vi "formate date.vi"(9 "Sepertaor":string, 10 "Input Date":string, 11 "Layout":string(combo)="[MMM-YYYY]") -> (2 "Formatted Date":string)   [LabVIEW 2015]
panel:
  in  "error in (no error)":errorcluster
  out "error IO":errorcluster
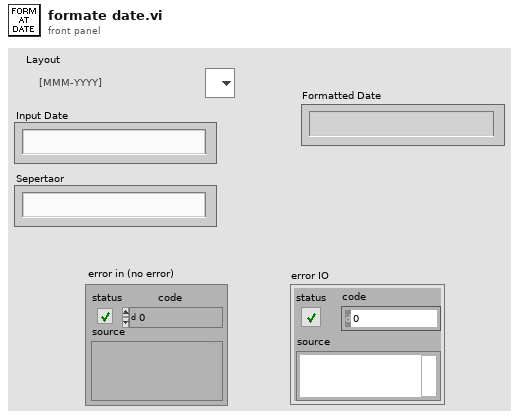
[diagram p1: front panel]
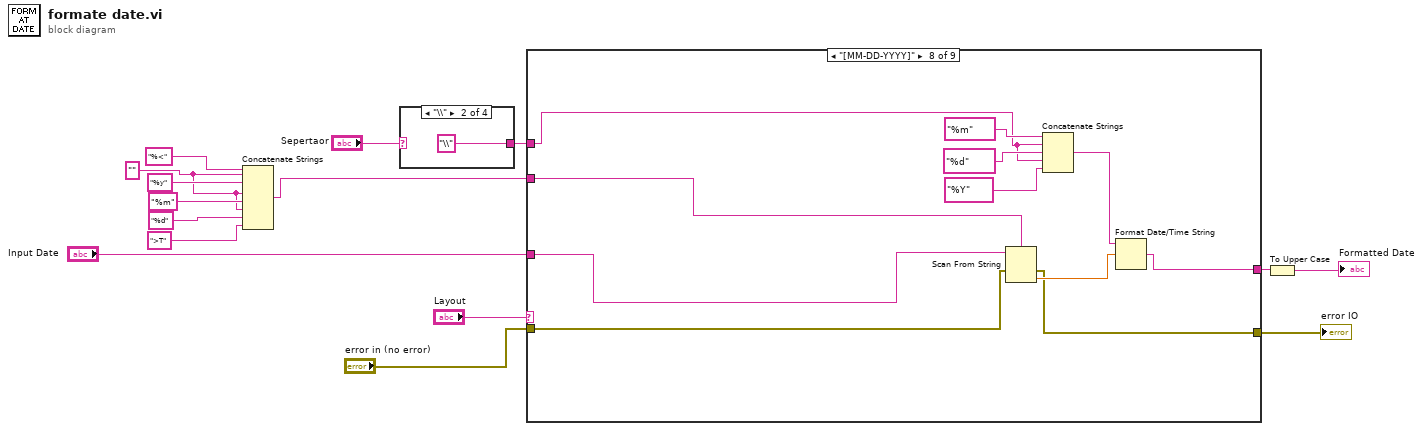
[diagram p0: block diagram]
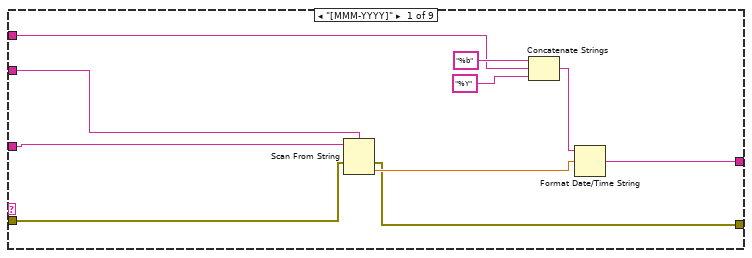
[diagram p2: hidden frame]
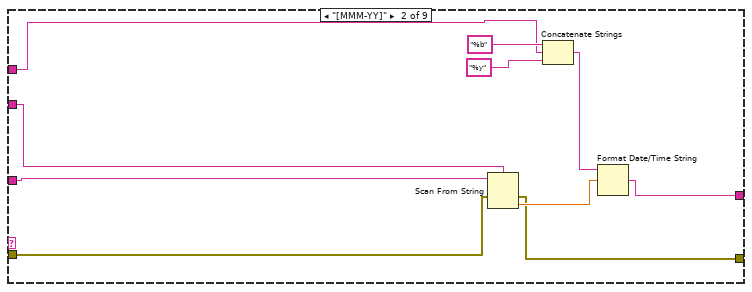
[diagram p3: hidden frame]
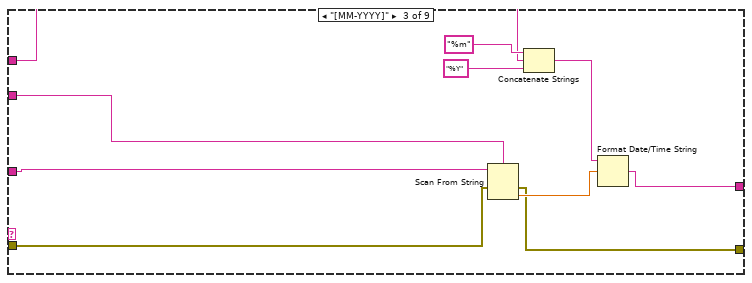
[diagram p4: hidden frame]
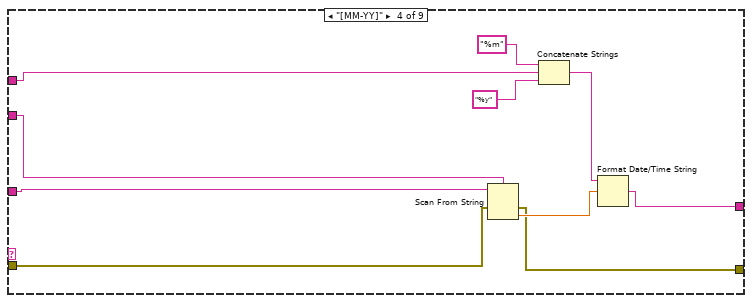
[diagram p5: hidden frame]
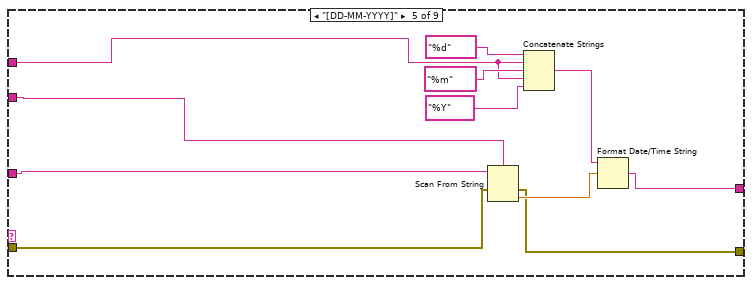
[diagram p6: hidden frame]
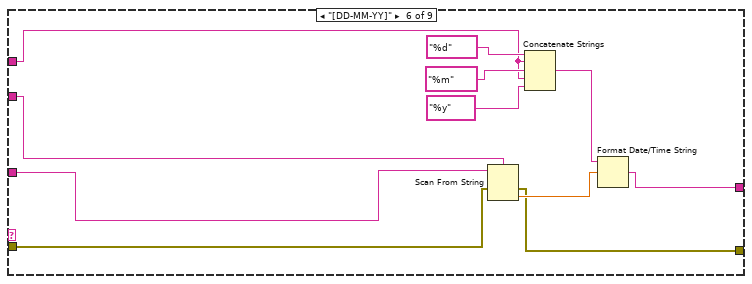
[diagram p7: hidden frame]
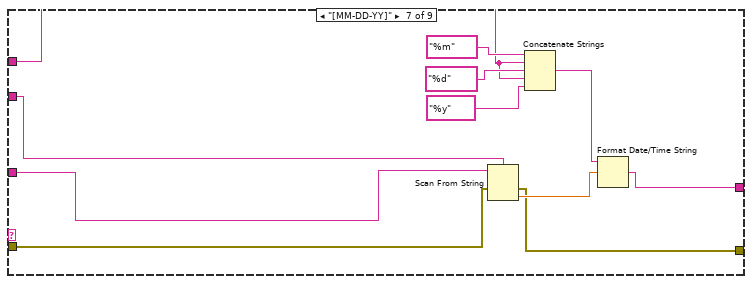
[diagram p8: hidden frame]
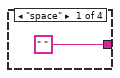
[diagram p10: hidden frame]
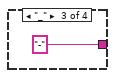
[diagram p11: hidden frame]
diagram:
  w10 = "" ("Sepertaor")
  n1 = Concatenate Strings("%<" ("string"), w10, "%y" ("string"), w10, "%m" ("string"), w10, "%d" ("string"), ">T" ("string")) -> (w9:string)
  n2 = case shown="\"\\\\\"" "Sepertaor" {
    selector: "Sepertaor" -> [_ _ _ w19]
    tunnel: [" " "\\" "-" w19] -> w1
    frame "space" {
    }
    frame "\\" {
    }
    frame "_" {
    }
    frame Default {
    }
  }
  n3 = case shown="\"[MM-DD-YYYY]\"" "Layout" {
    tunnel: [w26 w36 w46 w56 w67 w79 w90 w101 w104] -> w3
    tunnel: "Input Date" -> [w29 w39 w49 w59 w70 w73 w84 w95 w104]
    tunnel: "error in (no error)" -> [w25 w35 w45 w55 w66 w78 w89 w100 _]
    tunnel: [w27 w37 w47 w57 w68 w80 w91 w102 _] -> w6
    tunnel: w1 -> [w21 w31 w41 w51 w61 w72 w83 w94 _]
    tunnel: w9 -> [w20 w30 w40 w50 w60 w71 w82 w93 _]
    frame "[MMM-YYYY]" {
      n4 = Scan From String(format string=w20, input string=w29, error in=w25) -> (error out=w27:errorcluster, output 1=w28:dbl)  [unwired: 2 in, 2 out]
      n5 = Concatenate Strings("%b" ("time format string (%c)"), w21, "%Y" ("time format string (%c)")) -> (w22:string)
      n6 = Format Date/Time String(time format string (%c)=w22, seconds (now)=w28) -> (date/time string=w26:string)  [unwired: 1 in]
    }
    frame "[MMM-YY]" {
      n7 = Scan From String(format string=w30, input string=w39, error in=w35) -> (error out=w37:errorcluster, output 1=w38:dbl)  [unwired: 2 in, 2 out]
      n8 = Concatenate Strings("%b" ("time format string (%c)"), w31, "%y" ("time format string (%c)")) -> (w32:string)
      n9 = Format Date/Time String(time format string (%c)=w32, seconds (now)=w38) -> (date/time string=w36:string)  [unwired: 1 in]
    }
    frame "[MM-YYYY]" {
      n10 = Scan From String(format string=w40, input string=w49, error in=w45) -> (error out=w47:errorcluster, output 1=w48:dbl)  [unwired: 2 in, 2 out]
      n11 = Concatenate Strings("%m" ("time format string (%c)"), w41, "%Y" ("time format string (%c)")) -> (w43:string)
      n12 = Format Date/Time String(time format string (%c)=w43, seconds (now)=w48) -> (date/time string=w46:string)  [unwired: 1 in]
    }
    frame "[MM-YY]" {
      n13 = Scan From String(format string=w50, input string=w59, error in=w55) -> (error out=w57:errorcluster, output 1=w58:dbl)  [unwired: 2 in, 2 out]
      n14 = Concatenate Strings("%m" ("time format string (%c)"), w51, "%y" ("time format string (%c)")) -> (w53:string)
      n15 = Format Date/Time String(time format string (%c)=w53, seconds (now)=w58) -> (date/time string=w56:string)  [unwired: 1 in]
    }
    frame "[DD-MM-YYYY]" {
      n16 = Scan From String(format string=w60, input string=w70, error in=w66) -> (error out=w68:errorcluster, output 1=w69:dbl)  [unwired: 2 in, 2 out]
      n17 = Concatenate Strings("%d" ("time format string (%c)"), w61, "%m" ("time format string (%c)"), w61, "%Y" ("time format string (%c)")) -> (w64:string)
      n18 = Format Date/Time String(time format string (%c)=w64, seconds (now)=w69) -> (date/time string=w67:string)  [unwired: 1 in]
    }
    frame "[DD-MM-YY]" {
      n19 = Scan From String(format string=w71, input string=w73, error in=w78) -> (error out=w80:errorcluster, output 1=w81:dbl)  [unwired: 2 in, 2 out]
      n20 = Concatenate Strings("%d" ("time format string (%c)"), w72, "%m" ("time format string (%c)"), w72, "%y" ("time format string (%c)")) -> (w76:string)
      n21 = Format Date/Time String(time format string (%c)=w76, seconds (now)=w81) -> (date/time string=w79:string)  [unwired: 1 in]
    }
    frame "[MM-DD-YY]" {
      n22 = Scan From String(format string=w82, input string=w84, error in=w89) -> (error out=w91:errorcluster, output 1=w92:dbl)  [unwired: 2 in, 2 out]
      n23 = Concatenate Strings("%m" ("time format string (%c)"), w83, "%d" ("time format string (%c)"), w83, "%y" ("time format string (%c)")) -> (w87:string)
      n24 = Format Date/Time String(time format string (%c)=w87, seconds (now)=w92) -> (date/time string=w90:string)  [unwired: 1 in]
    }
    frame "[MM-DD-YYYY]" {
      n25 = Scan From String(format string=w93, input string=w95, error in=w100) -> (error out=w102:errorcluster, output 1=w103:dbl)  [unwired: 2 in, 2 out]
      n26 = Concatenate Strings("%m" ("time format string (%c)"), w94, "%d" ("time format string (%c)"), w94, "%Y" ("time format string (%c)")) -> (w98:string)
      n27 = Format Date/Time String(time format string (%c)=w98, seconds (now)=w103) -> (date/time string=w101:string)  [unwired: 1 in]
    }
    frame Default {
    }
  }
  "error IO" <- w6
  n28 = To Upper Case(1:w3) -> (0:→"Formatted Date":string)
